vi "temp control global variables.vi"() -> ()   [LabVIEW 2016]
doc: "These are the global variables for the temperature control system including:\n\n1) The HP34401A globals\n2) The PID globals\n3) The Temp controller globals\n\nPaul K Dixon\nPhysics 350\nCSUSB Physics"
uses:
  typedefs/control parameters.ctl
  typedefs/scale control.ctl
panel:
  in  "T cont exited":bool
  in  "exit T cont":bool
  in  "Scale Control":T1
  out "settled":bool
  in  "Control Parameters":T2={"Setpoint"=30.0, "Control bandwidth"=4.0, "Settle bandwidth"=1.0, "Integral time"=30.0, "Int\non"=TRUE, "Derivative time"=0.5, "Der\non"=TRUE, "Settle time"=30.0} {"Settle time" format="%.2f"; "Derivative time" format="%.2f"; "Integral time" format="%.2f"; "Settle bandwidth" format="%.2f"; "Control bandwidth" format="%.2f"; "Setpoint" format="%.2f"}
  in  "Reset PID (auto clear)":bool
  # "Temp Chart Global Variables"
  # "PID Global Variables"
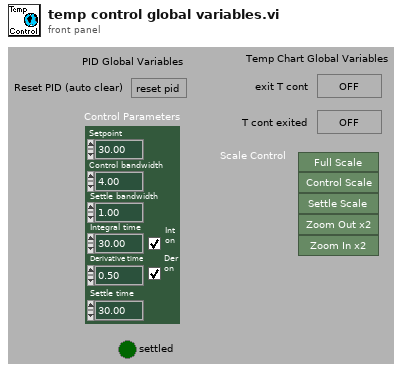
[diagram p1: front panel]
types:
  T1 = typedef "scale control.ctl" = cluster{"Full Scale":bool, "Control Scale":bool, "Settle Scale":bool, "Zoom Out":bool, "Zoom In":bool}
  T2 = typedef "control parameters.ctl" = cluster{"Setpoint":dbl, "Control bandwidth":dbl, "Settle bandwidth":dbl, "Integral time":dbl, "Int\non":bool, "Derivative time":dbl, "Der\non":bool, "Settle time":dbl}
diagram:
